vi "Read SS with Header.vi"(0 "file path":path, 11 "Transpose Data Array":bool, 13 "use int dialog (default=T)":bool=TRUE) -> (4 "Header String":string, 8 "Data Read":dbl[][](array[numeric]) format="%.2f", 15 "cancelled":bool)   [LabVIEW 2019]
doc: "This vi reads a 2D spreadsheet and a text header from a file. It is meant to work specifically with Write SS with Header.vi\n\nThe parser string is [CR, CR, \"<data below>\", CR, CR].\n\nThe error handling is embedded.\n\nPaul K Dixon\nP3600\nCSUSB Physics"
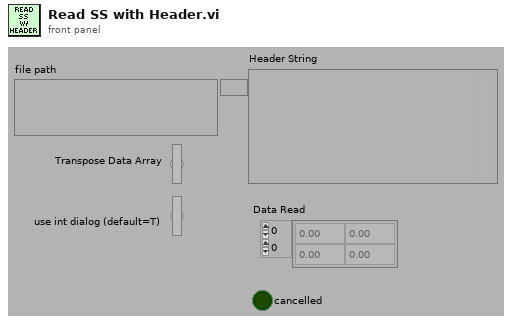
[diagram p1: front panel]
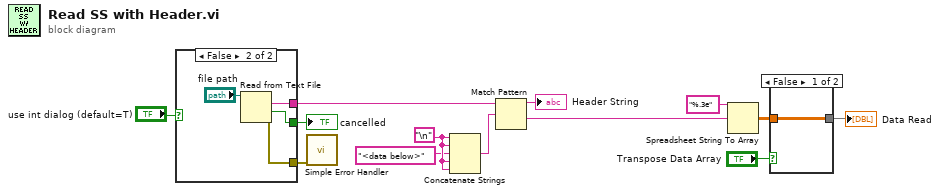
[diagram p0: block diagram]
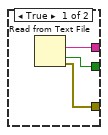
[diagram p2: hidden frame]
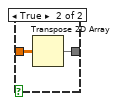
[diagram p3: hidden frame]
diagram:
  w6 = "\n"
  n1 = case shown="False" "use int dialog (default=T)" {
    tunnel: [w16 w20] -> w4
    tunnel: [w14 w18] -> w2
    tunnel: [w15 w17] -> w1
    frame True {
      n2 = Read from Text File() -> (text=w16:string, cancelled=w15:bool, error out=w14:errorcluster)  [unwired: 4 in, 1 out]
    }
    frame False {
      n3 = Read from Text File(file (use dialog)="file path") -> (text=w20:string, cancelled=w17:bool, error out=w18:errorcluster)  [unwired: 3 in, 1 out]
    }
  }
  "cancelled" <- w1
  n4 = call <vilib>:"Simple Error Handler.vi"("error in (no error)"=w2) -> ()  [unwired: 4 in, 5 out]
  n5 = Concatenate Strings(w6, w6, "<data below>", w6, w6) -> (w13:string)
  n6 = Match Pattern(string=w4, regular expression=w13) -> (before substring=→"Header String":string, after substring=w11:string)  [unwired: 1 in, 2 out]
  n7 = Spreadsheet String To Array(format string="%.3e", spreadsheet string=w11) -> (array=w9:dbl[][])  [unwired: 2 in]
  n8 = case shown="False" "Transpose Data Array" {
    tunnel: w9 -> [w21 w23]
    tunnel: [w21 w22] -> w7
    frame False {
    }
    frame True {
      n9 = Transpose 2D Array(2D array=w23) -> (transposed array=w22:dbl[][])
    }
  }
  "Data Read" <- w7
